vi "rsidr_core_global.vi"() -> ()   [LabVIEW 2020, in "Rohde&Schwarz CMWXP NR FR1 Measurement.lvlib"] (continued)
{"Level"=4, "Class Only"=FALSE, "Identifier"="RSCMWXPNRFR1M_ATTR_FETCH_MULTI_EVAL_MEAS_ACLR_CURRENT_RESULTS", "Descriptive Name"="Fetch Multi Eval Meas ACLR Current Results", "Data Type"=enum."RawString", "Command"="FETC:NRS:MEAS{instance}:MEV:ACLR:CURR?", "Access"=enum."Read Only", "Range Table"="", "Read Callback"="", "Write Callback"="", "Range Callback"="", "Check Callback"="", "Rngtable Callback"="", "Coerce Callback"="", "Supported Models"="", "Instrument Options"="", "Check Status Callback"="", "Flags"=0, "Help"="Returns the relative ACLR values for NR standalone, as displayed in the table below the ACLR diagram. The current values are retrieved.\n\nReturn values:  \n<Reliability>\n decimal\n\n<UTRA2neg>\n float\nACLR for the second UTRA channel with lower frequency\nDefault unit:  dB \n\n<UTRA1neg>\n float\nACLR for the first UTRA channel with lower frequency\nDefault unit:  dB \n\n<NRneg>\n float\nACLR for the first NR channel with lower frequency\nDefault unit:  dB \n\n<Carrier>\n float\nPower in the allocated NR channel\nDefault unit:  dBm \n\n<NRpos>\n float\nACLR for the first NR channel with higher frequency\nDefault unit:  dB \n\n<UTRA1pos>\n float\nACLR for the first UTRA channel with higher frequency\nDefault unit:  dB \n\n<UTRA2pos>\n float\nACLR for the second UTRA channel with higher frequency\nDefault unit:  dB\n\nAvailable Repeated Capabilities:\ninstance: i0, i1, i2, i3, i4, i5, i6, i7, i8, i9, i10, i11, i12, i13, i14, i15, i16, i17, i18, i19, i20, i21, i22, i23, i24, i25, i26, i27, i28, i29, i30, i31, i32\r\n\nRemote-control command(s):\nFETCh:NRSub:MEAS<i>:MEValuation:ACLR:CURRent?"}, {"Level"=4, "Class Only"=FALSE, "Identifier"="RSCMWXPNRFR1M_ATTR_FETCH_MULTI_EVAL_MEAS_ACLR_AVERAGE_RESULTS", "Descriptive Name"="Fetch Multi Eval Meas ACLR Average Results", "Data Type"=enum."RawString", "Command"="FETC:NRS:MEAS{instance}:MEV:ACLR:AVER?", "Access"=enum."Read Only", "Range Table"="", "Read Callback"="", "Write Callback"="", "Range Callback"="", "Check Callback"="", "Rngtable Callback"="", "Coerce Callback"="", "Supported Models"="", "Instrument Options"="", "Check Status Callback"="", "Flags"=0, "Help"="Returns the relative ACLR values for NR standalone, as displayed in the table below the ACLR diagram. The average values are retrieved.\n\nReturn values:  \n<Reliability>\n decimal\n\n<UTRA2neg>\n float\nACLR for the second UTRA channel with lower frequency\nDefault unit:  dB \n\n<UTRA1neg>\n float\nACLR for the first UTRA channel with lower frequency\nDefault unit:  dB \n\n<NRneg>\n float\nACLR for the first NR channel with lower frequency\nDefault unit:  dB \n\n<Carrier>\n float\nPower in the allocated NR channel\nDefault unit:  dBm \n\n<NRpos>\n float\nACLR for the first NR channel with higher frequency\nDefault unit:  dB \n\n<UTRA1pos>\n float\nACLR for the first UTRA channel with higher frequency\nDefault unit:  dB \n\n<UTRA2pos>\n float\nACLR for the second UTRA channel with higher frequency\nDefault unit:  dB\n\nAvailable Repeated Capabilities:\ninstance: i0, i1, i2, i3, i4, i5, i6, i7, i8, i9, i10, i11, i12, i13, i14, i15, i16, i17, i18, i19, i20, i21, i22, i23, i24, i25, i26, i27, i28, i29, i30, i31, i32\r\n\nRemote-control command(s):\nFETCh:NRSub:MEAS<i>:MEValuation:ACLR:AVERage?"}, {"Level"=4, "Class Only"=FALSE, "Identifier"="RSCMWXPNRFR1M_ATTR_QUERY_MULTI_EVAL_MEAS_ACLR_CURRENT_LIMIT_CHECK_RESULTS", "Descriptive Name"="Query Multi Eval Meas ACLR Current Limit Check Results", "Data Type"=enum."RawString", "Command"="CALC:NRS:MEAS{instance}:MEV:ACLR:CURR?", "Access"=enum."Read Only", "Range Table"="", "Read Callback"="", "Write Callback"="", "Range Callback"="", "Check Callback"="", "Rngtable Callback"="", "Coerce Callback"="", "Supported Models"="", "Instrument Options"="", "Check Status Callback"="", "Flags"=0, "Help"="Returns the limit check ACLR values for NR standalone, as displayed in the table below the ACLR diagram. The current values are used.\n\nReturn values:  \n<Reliability>\n decimal\n\n<UTRA2negLimCheck>\n limit check result\nLimit check result for the second UTRA channel with lower frequency\n\n<UTRA1negLimCheck>\n limit check result\nLimit check result for the first UTRA channel with lower frequency\n\n<NRnegLimCheck>\n limit check result\nLimit check result for the first NR channel with lower frequency\n\n<CarrierLimCheck>\n limit check result\nLimit check result for power in the allocated NR channel\n\n<NRposLimCheck>\n limit check result\nLimit check result for the first NR channel with higher frequency\n\n<UTRA1posLimCheck>\n limit check result\nLimit check result for the first UTRA channel with higher frequency\n\n<UTRA2posLimCheck>\n limit check result\nLimit check result for the second UTRA channel with higher frequency\n\nAvailable Repeated Capabilities:\ninstance: i0, i1, i2, i3, i4, i5, i6, i7, i8, i9, i10, i11, i12, i13, i14, i15, i16, i17, i18, i19, i20, i21, i22, i23, i24, i25, i26, i27, i28, i29, i30, i31, i32\r\n\nRemote-control command(s):\nCALCulate:NRSub:MEAS<i>:MEValuation:ACLR:CURRent?"}, {"Level"=4, "Class Only"=FALSE, "Identifier"="RSCMWXPNRFR1M_ATTR_QUERY_MULTI_EVAL_MEAS_ACLR_AVERAGE_LIMIT_CHECK_RESULTS", "Descriptive Name"="Query Multi Eval Meas ACLR Average Limit Check Results", "Data Type"=enum."RawString", "Command"="CALC:NRS:MEAS{instance}:MEV:ACLR:AVER?", "Access"=enum."Read Only", "Range Table"="", "Read Callback"="", "Write Callback"="", "Range Callback"="", "Check Callback"="", "Rngtable Callback"="", "Coerce Callback"="", "Supported Models"="", "Instrument Options"="", "Check Status Callback"="", "Flags"=0, "Help"="Returns the limit check ACLR values for NR standalone, as displayed in the table below the ACLR diagram. The average values are used.\n\nReturn values:  \n<Reliability>\n decimal\n\n<UTRA2negLimCheck>\n limit check result\nLimit check result for the second UTRA channel with lower frequency\n\n<UTRA1negLimCheck>\n limit check result\nLimit check result for the first UTRA channel with lower frequency\n\n<NRnegLimCheck>\n limit check result\nLimit check result for the first NR channel with lower frequency\n\n<CarrierLimCheck>\n limit check result\nLimit check result for power in the allocated NR channel\n\n<NRposLimCheck>\n limit check result\nLimit check result for the first NR channel with higher frequency\n\n<UTRA1posLimCheck>\n limit check result\nLimit check result for the first UTRA channel with higher frequency\n\n<UTRA2posLimCheck>\n limit check result\nLimit check result for the second UTRA channel with higher frequency\n\nAvailable Repeated Capabilities:\ninstance: i0, i1, i2, i3, i4, i5, i6, i7, i8, i9, i10, i11, i12, i13, i14, i15, i16, i17, i18, i19, i20, i21, i22, i23, i24, i25, i26, i27, i28, i29, i30, i31, i32\r\n\nRemote-control command(s):\nCALCulate:NRSub:MEAS<i>:MEValuation:ACLR:AVERage?"}, {"Level"=4, "Class Only"=FALSE, "Identifier"="RSCMWXPNRFR1M_ATTR_READ_MULTI_EVAL_MEAS_ACLR_ENDC_CURRENT_RESULTS", "Descriptive Name"="Read Multi Eval Meas ACLR EN-DC Current Results", "Data Type"=enum."RawString", "Command"="READ:NRS:MEAS{instance}:MEV:ACLR:ENDC:CURR?", "Access"=enum."Read Only", "Range Table"="", "Read Callback"="", "Write Callback"="", "Range Callback"="", "Check Callback"="", "Rngtable Callback"="", "Coerce Callback"="", "Supported Models"="", "Instrument Options"="", "Check Status Callback"="", "Flags"=0, "Help"="Returns the relative ACLR values for EN-DC, as displayed in the table below the ACLR diagram. The current values are retrieved.\n\nReturn values:  \n<Reliability>\n decimal\n\n<ENDCneg>\n float\nACLR for the adjacent channel with lower frequency\nDefault unit:  dB \n\n<Carrier>\n float\nPower in the allocated channel (aggregated BW)\nDefault unit:  dBm \n\n<ENDCpos>\n float\nACLR for the adjacent channel with higher frequency\nDefault unit:  dB\n\nAvailable Repeated Capabilities:\ninstance: i0, i1, i2, i3, i4, i5, i6, i7, i8, i9, i10, i11, i12, i13, i14, i15, i16, i17, i18, i19, i20, i21, i22, i23, i24, i25, i26, i27, i28, i29, i30, i31, i32\r\n\nRemote-control command(s):\nREAD:NRSub:MEAS<i>:MEValuation:ACLR:ENDC:CURRent?"}, {"Level"=4, "Class Only"=FALSE, "Identifier"="RSCMWXPNRFR1M_ATTR_READ_MULTI_EVAL_MEAS_ACLR_ENDC_AVERAGE_RESULTS", "Descriptive Name"="Read Multi Eval Meas ACLR EN-DC Average Results", "Data Type"=enum."RawString", "Command"="READ:NRS:MEAS{instance}:MEV:ACLR:ENDC:AVER?", "Access"=enum."Read Only", "Range Table"="", "Read Callback"="", "Write Callback"="", "Range Callback"="", "Check Callback"="", "Rngtable Callback"="", "Coerce Callback"="", "Supported Models"="", "Instrument Options"="", "Check Status Callback"="", "Flags"=0, "Help"="Returns the relative ACLR values for EN-DC, as displayed in the table below the ACLR diagram. The average values are retrieved.\n\nReturn values:  \n<Reliability>\n decimal\n\n<ENDCneg>\n float\nACLR for the adjacent channel with lower frequency\nDefault unit:  dB \n\n<Carrier>\n float\nPower in the allocated channel (aggregated BW)\nDefault unit:  dBm \n\n<ENDCpos>\n float\nACLR for the adjacent channel with higher frequency\nDefault unit:  dB\n\nAvailable Repeated Capabilities:\ninstance: i0, i1, i2, i3, i4, i5, i6, i7, i8, i9, i10, i11, i12, i13, i14, i15, i16, i17, i18, i19, i20, i21, i22, i23, i24, i25, i26, i27, i28, i29, i30, i31, i32\r\n\nRemote-control command(s):\nREAD:NRSub:MEAS<i>:MEValuation:ACLR:ENDC:AVERage?"}, {"Level"=4, "Class Only"=FALSE, "Identifier"="RSCMWXPNRFR1M_ATTR_FETCH_MULTI_EVAL_MEAS_ACLR_ENDC_CURRENT_RESULTS", "Descriptive Name"="Fetch Multi Eval Meas ACLR EN-DC Current Results", "Data Type"=enum."RawString", "Command"="FETC:NRS:MEAS{instance}:MEV:ACLR:ENDC:CURR?", "Access"=enum."Read Only", "Range Table"="", "Read Callback"="", "Write Callback"="", "Range Callback"="", "Check Callback"="", "Rngtable Callback"="", "Coerce Callback"="", "Supported Models"="", "Instrument Options"="", "Check Status Callback"="", "Flags"=0, "Help"="Returns the relative ACLR values for EN-DC, as displayed in the table below the ACLR diagram. The current values are retrieved.\n\nReturn values:  \n<Reliability>\n decimal\n\n<ENDCneg>\n float\nACLR for the adjacent channel with lower frequency\nDefault unit:  dB \n\n<Carrier>\n float\nPower in the allocated channel (aggregated BW)\nDefault unit:  dBm \n\n<ENDCpos>\n float\nACLR for the adjacent channel with higher frequency\nDefault unit:  dB\n\nAvailable Repeated Capabilities:\ninstance: i0, i1, i2, i3, i4, i5, i6, i7, i8, i9, i10, i11, i12, i13, i14, i15, i16, i17, i18, i19, i20, i21, i22, i23, i24, i25, i26, i27, i28, i29, i30, i31, i32\r\n\nRemote-control command(s):\nFETCh:NRSub:MEAS<i>:MEValuation:ACLR:ENDC:CURRent?"}, {"Level"=4, "Class Only"=FALSE, "Identifier"="RSCMWXPNRFR1M_ATTR_FETCH_MULTI_EVAL_MEAS_ACLR_ENDC_AVERAGE_RESULTS", "Descriptive Name"="Fetch Multi Eval Meas ACLR EN-DC Average Results", "Data Type"=enum."RawString", "Command"="FETC:NRS:MEAS{instance}:MEV:ACLR:ENDC:AVER?", "Access"=enum."Read Only", "Range Table"="", "Read Callback"="", "Write Callback"="", "Range Callback"="", "Check Callback"="", "Rngtable Callback"="", "Coerce Callback"="", "Supported Models"="", "Instrument Options"="", "Check Status Callback"="", "Flags"=0, "Help"="Returns the relative ACLR values for EN-DC, as displayed in the table below the ACLR diagram. The average values are retrieved.\n\nReturn values:  \n<Reliability>\n decimal\n\n<ENDCneg>\n float\nACLR for the adjacent channel with lower frequency\nDefault unit:  dB \n\n<Carrier>\n float\nPower in the allocated channel (aggregated BW)\nDefault unit:  dBm \n\n<ENDCpos>\n float\nACLR for the adjacent channel with higher frequency\nDefault unit:  dB\n\nAvailable Repeated Capabilities:\ninstance: i0, i1, i2, i3, i4, i5, i6, i7, i8, i9, i10, i11, i12, i13, i14, i15, i16, i17, i18, i19, i20, i21, i22, i23, i24, i25, i26, i27, i28, i29, i30, i31, i32\r\n\nRemote-control command(s):\nFETCh:NRSub:MEAS<i>:MEValuation:ACLR:ENDC:AVERage?"}, {"Level"=4, "Class Only"=FALSE, "Identifier"="RSCMWXPNRFR1M_ATTR_QUERY_MULTI_EVAL_MEAS_ACLR_ENDC_CURRENT_LIMIT_CHECK_RESULTS", "Descriptive Name"="Query Multi Eval Meas ACLR EN-DC Current Limit Check Results", "Data Type"=enum."RawString", "Command"="CALC:NRS:MEAS{instance}:MEV:ACLR:ENDC:CURR?", "Access"=enum."Read Only", "Range Table"="", "Read Callback"="", "Write Callback"="", "Range Callback"="", "Check Callback"="", "Rngtable Callback"="", "Coerce Callback"="", "Supported Models"="", "Instrument Options"="", "Check Status Callback"="", "Flags"=0, "Help"="Returns the ACLR limit check values for EN-DC, as displayed in the table below the ACLR diagram. The current values are used.\n\nReturn values:  \n<Reliability>\n decimal\n\n<ENDCnegLimCheck>\n limit check result\nLimit check result for the adjacent channel with lower frequency\n\n<CarrierLimCheck>\n limit check result\nLimit check result for power in the allocated channel (aggregated BW)\n\n<ENDCposLimCheck>\n limit check result\nLimit check result for the adjacent channel with higher frequency\n\nAvailable Repeated Capabilities:\ninstance: i0, i1, i2, i3, i4, i5, i6, i7, i8, i9, i10, i11, i12, i13, i14, i15, i16, i17, i18, i19, i20, i21, i22, i23, i24, i25, i26, i27, i28, i29, i30, i31, i32\r\n\nRemote-control command(s):\nCALCulate:NRSub:MEAS<i>:MEValuation:ACLR:ENDC:CURRent?"}, {"Level"=4, "Class Only"=FALSE, "Identifier"="RSCMWXPNRFR1M_ATTR_QUERY_MULTI_EVAL_MEAS_ACLR_ENDC_AVERAGE_LIMIT_CHECK_RESULTS", "Descriptive Name"="Query Multi Eval Meas ACLR EN-DC Average Limit Check Results", "Data Type"=enum."RawString", "Command"="CALC:NRS:MEAS{instance}:MEV:ACLR:ENDC:AVER?", "Access"=enum."Read Only", "Range Table"="", "Read Callback"="", "Write Callback"="", "Range Callback"="", "Check Callback"="", "Rngtable Callback"="", "Coerce Callback"="", "Supported Models"="", "Instrument Options"="", "Check Status Callback"="", "Flags"=0, "Help"="Returns the ACLR limit check values for EN-DC, as displayed in the table below the ACLR diagram. The current values are used.\n\nReturn values:  \n<Reliability>\n decimal\n\n<ENDCnegLimCheck>\n limit check result\nLimit check result for the adjacent channel with lower frequency\n\n<CarrierLimCheck>\n limit check result\nLimit check result for power in the allocated channel (aggregated BW)\n\n<ENDCposLimCheck>\n limit check result\nLimit check result for the adjacent channel with higher frequency\n\nAvailable Repeated Capabilities:\ninstance: i0, i1, i2, i3, i4, i5, i6, i7, i8, i9, i10, i11, i12, i13, i14, i15, i16, i17, i18, i19, i20, i21, i22, i23, i24, i25, i26, i27, i28, i29, i30, i31, i32\r\n\nRemote-control command(s):\nCALCulate:NRSub:MEAS<i>:MEValuation:ACLR:ENDC:AVERage?"}, {"Level"=3, "Class Only"=TRUE, "Identifier"="", "Descriptive Name"="IQ Constellation", "Data Type"=enum."ViInt32", "Command"="", "Access"=enum."Read Only", "Range Table"="", "Read Callback"="", "Write Callback"="", "Range Callback"="", "Check Callback"="", "Rngtable Callback"="", "Coerce Callback"="", "Supported Models"="", "Instrument Options"="", "Check Status Callback"="", "Flags"=0, "Help"="This class contains commands that return the contents of the I/Q constellation diagram."}, {"Level"=4, "Class Only"=FALSE, "Identifier"="RSCMWXPNRFR1M_ATTR_FETCH_MULTI_EVAL_MEAS_TRACE_IQ_CONSTELLATION_LOW_RESULTS", "Descriptive Name"="Fetch Multi Eval Meas Trace IQ Constellation Low Results", "Data Type"=enum."RawString", "Command"="FETC:NRS:MEAS{instance}:MEV:TRAC:IQ:LOW?", "Access"=enum."Read Only", "Range Table"="", "Read Callback"="", "Write Callback"="", "Range Callback"="", "Check Callback"="", "Rngtable Callback"="", "Coerce Callback"="", "Supported Models"="", "Instrument Options"="", "Check Status Callback"="", "Flags"=0, "Help"="Returns the results in the I/Q constellation diagram for low EVM window position.\n\nThere is one pair of values per modulation symbol. The results are returned in the following order:\n<Reliability>, {<IPhase>, <QPhase>}symbol 1, ..., {<IPhase>, <QPhase>}symbol n\n\nReturn values:  \n<Reliability>\n decimal\n\n<IPhase>\n float\nNormalized I amplitude\n\n<QPhase>\n float\nNormalized Q amplitude\n\nAvailable Repeated Capabilities:\ninstance: i0, i1, i2, i3, i4, i5, i6, i7, i8, i9, i10, i11, i12, i13, i14, i15, i16, i17, i18, i19, i20, i21, i22, i23, i24, i25, i26, i27, i28, i29, i30, i31, i32\r\n\nRemote-control command(s):\nFETCh:NRSub:MEAS<i>:MEValuation:TRACe:IQ:LOW?"}, {"Level"=4, "Class Only"=FALSE, "Identifier"="RSCMWXPNRFR1M_ATTR_FETCH_MULTI_EVAL_MEAS_TRACE_IQ_CONSTELLATION_HIGH_RESULTS", "Descriptive Name"="Fetch Multi Eval Meas Trace IQ Constellation High Results", "Data Type"=enum."RawString", "Command"="FETC:NRS:MEAS{instance}:MEV:TRAC:IQ:HIGH?", "Access"=enum."Read Only", "Range Table"="", "Read Callback"="", "Write Callback"="", "Range Callback"="", "Check Callback"="", "Rngtable Callback"="", "Coerce Callback"="", "Supported Models"="", "Instrument Options"="", "Check Status Callback"="", "Flags"=0, "Help"="Returns the results in the I/Q constellation diagram for high EVM window position.\n\nThere is one pair of values per modulation symbol. The results are returned in the following order:\n<Reliability>, {<IPhase>, <QPhase>}symbol 1, ..., {<IPhase>, <QPhase>}symbol n\n\nReturn values:  \n<Reliability>\n decimal\n\n<IPhase>\n float\nNormalized I amplitude\n\n<QPhase>\n float\nNormalized Q amplitude\n\nAvailable Repeated Capabilities:\ninstance: i0, i1, i2, i3, i4, i5, i6, i7, i8, i9, i10, i11, i12, i13, i14, i15, i16, i17, i18, i19, i20, i21, i22, i23, i24, i25, i26, i27, i28, i29, i30, i31, i32\r\n\nRemote-control command(s):\nFETCh:NRSub:MEAS<i>:MEValuation:TRACe:IQ:HIGH?"}, {"Level"=3, "Class Only"=TRUE, "Identifier"="", "Descriptive Name"="Modulation", "Data Type"=enum."ViInt32", "Command"="", "Access"=enum."Read Only", "Range Table"="", "Read Callback"="", "Write Callback"="", "Range Callback"="", "Check Callback"="", "Rngtable Callback"="", "Coerce Callback"="", "Supported Models"="", "Instrument Options"="", "Check Status Callback"="", "Flags"=0, "Help"="The commands in this class return the statistical modulation results."}, {"Level"=4, "Class Only"=FALSE, "Identifier"="RSCMWXPNRFR1M_ATTR_READ_MULTI_EVAL_MEAS_MODULATION_CURRENT_RESULTS", "Descriptive Name"="Read Multi Eval Meas Modulation Current Results", "Data Type"=enum."RawString", "Command"="READ:NRS:MEAS{instance}:MEV:MOD:CURR?", "Access"=enum."Read Only", "Range Table"="", "Read Callback"="", "Write Callback"="", "Range Callback"="", "Check Callback"="", "Rngtable Callback"="", "Coerce Callback"="", "Supported Models"="", "Instrument Options"="", "Check Status Callback"="", "Flags"=0, "Help"="Return the current single value results.\n\nReturn values:  \n<1_Reliability>\n decimal\n\n<2_OutOfTol>\n decimal\nOut of tolerance result, i.e. percentage of measurement intervals of the statistic count for modulation measurements exceeding the specified modulation limits.\nDefault unit:  % \n\n<3_EVM_RMSlow>\n float\nEVM RMS value, low EVM window position\nDefault unit:  % \n\n<4_EVM_RMShigh>\n float\nEVM RMS value, high EVM window position\nDefault unit:  % \n\n<5_EVMpeakLow>\n float\nEVM peak value, low EVM window position\nDefault unit:  % \n\n<6_EVMpeakHigh>\n float\nEVM peak value, high EVM window position\nDefault unit:  % \n\n<7_MErr_RMSlow>\n float\nMagnitude error RMS value, low EVM window position\nDefault unit:  % \n\n<8_MErr_RMShigh>\n float\nMagnitude error RMS value, high EVM window position\nDefault unit:  % \n\n<9_MErrPeakLow>\n float\nMagnitude error peak value, low EVM window position\nDefault unit:  % \n\n<10_MErrPeakHigh>\n float\nMagnitude error peak value, high EVM window position\nDefault unit:  % \n\n<11_PErr_RMSlow>\n float\nPhase error RMS value, low EVM window position\nDefault unit:  deg \n\n<12_PErr_RMSh>\n float\nPhase error RMS value, high EVM window position\nDefault unit:  deg \n\n<13_PErrPeakLow>\n float\nPhase error peak value, low EVM window position\nDefault unit:  deg \n\n<14_PErrPeakHigh>\n float\nPhase error peak value, high EVM window position\nDefault unit:  deg \n\n<15_IQoffset>\n float\nI/Q origin offset\nDefault unit:  dBc \n\n<16_FreqError>\n float\nCarrier frequency error\nDefault unit:  Hz \n\n<17_TimingError>\n float\nTransmit time error\nDefault unit:  Ts (basic time unit) \n\n<18_TXpower>\n float\nUser equipment power\nDefault unit:  dBm \n\n<19_PeakPower>\n float\nUser equipment peak power\nDefault unit:  dBm \n\n<20_RBpower>\n float\nRB power\nDefault unit:  dBm \n\n<21_EVM_DMRSl>\n float\nEVM DMRS value, low EVM window position\nDefault unit:  % \n\n<22_EVM_DMRSh>\n float\nEVM DMRS value, high EVM window position\nDefault unit:  % \n\n<23_MErr_DMRSl>\n float\nMagnitude error DMRS value, low EVM window position\nDefault unit:  % \n\n<24_MErr_DMRSh>\n float\nMagnitude error DMRS value, high EVM window position\nDefault unit:  % \n\n<25_PErr_DMRS>\n float\nPhase error DMRS value, low EVM window position\nDefault unit:  deg \n\n<26_PErr_DMRSh>\n float\nPhase error DMRS value, high EVM window position\nDefault unit:  deg \n\n<27_FreqErrorPpm>\n float\nCarrier frequency error in ppm\nDefault unit:  ppm \n\n<28_SampleClockE>\n float\nSample clock error\nDefault unit:  ppm\n\nAvailable Repeated Capabilities:\ninstance: i0, i1, i2, i3, i4, i5, i6, i7, i8, i9, i10, i11, i12, i13, i14, i15, i16, i17, i18, i19, i20, i21, i22, i23, i24, i25, i26, i27, i28, i29, i30, i31, i32\r\n\nRemote-control command(s):\nREAD:NRSub:MEAS<i>:MEValuation:MODulation:CURRent?"}, {"Level"=4, "Class Only"=FALSE, "Identifier"="RSCMWXPNRFR1M_ATTR_READ_MULTI_EVAL_MEAS_MODULATION_AVERAGE_RESULTS", "Descriptive Name"="Read Multi Eval Meas Modulation Average Results", "Data Type"=enum."RawString", "Command"="READ:NRS:MEAS{instance}:MEV:MOD:AVER?", "Access"=enum."Read Only", "Range Table"="", "Read Callback"="", "Write Callback"="", "Range Callback"="", "Check Callback"="", "Rngtable Callback"="", "Coerce Callback"="", "Supported Models"="", "Instrument Options"="", "Check Status Callback"="", "Flags"=0, "Help"="Return the average single value results.\n\nReturn values:  \n<1_Reliability>\n decimal\n\n<2_OutOfTol>\n decimal\nOut of tolerance result, i.e. percentage of measurement intervals of the statistic count for modulation measurements exceeding the specified modulation limits.\nDefault unit:  % \n\n<3_EVM_RMSlow>\n float\nEVM RMS value, low EVM window position\nDefault unit:  % \n\n<4_EVM_RMShigh>\n float\nEVM RMS value, high EVM window position\nDefault unit:  % \n\n<5_EVMpeakLow>\n float\nEVM peak value, low EVM window position\nDefault unit:  % \n\n<6_EVMpeakHigh>\n float\nEVM peak value, high EVM window position\nDefault unit:  % \n\n<7_MErr_RMSlow>\n float\nMagnitude error RMS value, low EVM window position\nDefault unit:  % \n\n<8_MErr_RMShigh>\n float\nMagnitude error RMS value, high EVM window position\nDefault unit:  % \n\n<9_MErrPeakLow>\n float\nMagnitude error peak value, low EVM window position\nDefault unit:  % \n\n<10_MErrPeakHigh>\n float\nMagnitude error peak value, high EVM window position\nDefault unit:  % \n\n<11_PErr_RMSlow>\n float\nPhase error RMS value, low EVM window position\nDefault unit:  deg \n\n<12_PErr_RMSh>\n float\nPhase error RMS value, high EVM window position\nDefault unit:  deg \n\n<13_PErrPeakLow>\n float\nPhase error peak value, low EVM window position\nDefault unit:  deg \n\n<14_PErrPeakHigh>\n float\nPhase error peak value, high EVM window position\nDefault unit:  deg \n\n<15_IQoffset>\n float\nI/Q origin offset\nDefault unit:  dBc \n\n<16_FreqError>\n float\nCarrier frequency error\nDefault unit:  Hz \n\n<17_TimingError>\n float\nTransmit time error\nDefault unit:  Ts (basic time unit) \n\n<18_TXpower>\n float\nUser equipment power\nDefault unit:  dBm \n\n<19_PeakPower>\n float\nUser equipment peak power\nDefault unit:  dBm \n\n<20_RBpower>\n float\nRB power\nDefault unit:  dBm \n\n<21_EVM_DMRSl>\n float\nEVM DMRS value, low EVM window position\nDefault unit:  % \n\n<22_EVM_DMRSh>\n float\nEVM DMRS value, high EVM window position\nDefault unit:  % \n\n<23_MErr_DMRSl>\n float\nMagnitude error DMRS value, low EVM window position\nDefault unit:  % \n\n<24_MErr_DMRSh>\n float\nMagnitude error DMRS value, high EVM window position\nDefault unit:  % \n\n<25_PErr_DMRS>\n float\nPhase error DMRS value, low EVM window position\nDefault unit:  deg \n\n<26_PErr_DMRSh>\n float\nPhase error DMRS value, high EVM window position\nDefault unit:  deg \n\n<27_FreqErrorPpm>\n float\nCarrier frequency error in ppm\nDefault unit:  ppm \n\n<28_SampleClockE>\n float\nSample clock error\nDefault unit:  ppm\n\nAvailable Repeated Capabilities:\ninstance: i0, i1, i2, i3, i4, i5, i6, i7, i8, i9, i10, i11, i12, i13, i14, i15, i16, i17, i18, i19, i20, i21, i22, i23, i24, i25, i26, i27, i28, i29, i30, i31, i32\r\n\nRemote-control command(s):\nREAD:NRSub:MEAS<i>:MEValuation:MODulation:AVERage?"}, {"Level"=4, "Class Only"=FALSE, "Identifier"="RSCMWXPNRFR1M_ATTR_READ_MULTI_EVAL_MEAS_MODULATION_STANDARD_DEVIATION_RESULTS", "Descriptive Name"="Read Multi Eval Meas Modulation Standard Deviation Results", "Data Type"=enum."RawString", "Command"="READ:NRS:MEAS{instance}:MEV:MOD:SDEV?", "Access"=enum."Read Only", "Range Table"="", "Read Callback"="", "Write Callback"="", "Range Callback"="", "Check Callback"="", "Rngtable Callback"="", "Coerce Callback"="", "Supported Models"="", "Instrument Options"="", "Check Status Callback"="", "Flags"=0, "Help"="Return the standard deviation single value results.\n\nReturn values:  \n<1_Reliability>\n decimal\n\n<2_OutOfTol>\n decimal\nOut of tolerance result, i.e. percentage of measurement intervals of the statistic count for modulation measurements exceeding the specified modulation limits.\nDefault unit:  % \n\n<3_EVM_RMSlow>\n float\nEVM RMS value, low EVM window position\nDefault unit:  % \n\n<4_EVM_RMShigh>\n float\nEVM RMS value, high EVM window position\nDefault unit:  % \n\n<5_EVMpeakLow>\n float\nEVM peak value, low EVM window position\nDefault unit:  % \n\n<6_EVMpeakHigh>\n float\nEVM peak value, high EVM window position\nDefault unit:  % \n\n<7_MErr_RMSlow>\n float\nMagnitude error RMS value, low EVM window position\nDefault unit:  % \n\n<8_MErr_RMShigh>\n float\nMagnitude error RMS value, high EVM window position\nDefault unit:  % \n\n<9_MErrPeakLow>\n float\nMagnitude error peak value, low EVM window position\nDefault unit:  % \n\n<10_MErrPeakHigh>\n float\nMagnitude error peak value, high EVM window position\nDefault unit:  % \n\n<11_PErr_RMSlow>\n float\nPhase error RMS value, low EVM window position\nDefault unit:  deg \n\n<12_PErr_RMSh>\n float\nPhase error RMS value, high EVM window position\nDefault unit:  deg \n\n<13_PErrPeakLow>\n float\nPhase error peak value, low EVM window position\nDefault unit:  deg \n\n<14_PErrPeakHigh>\n float\nPhase error peak value, high EVM window position\nDefault unit:  deg \n\n<15_IQoffset>\n float\nI/Q origin offset\nDefault unit:  dBc \n\n<16_FreqError>\n float\nCarrier frequency error\nDefault unit:  Hz \n\n<17_TimingError>\n float\nTransmit time error\nDefault unit:  Ts (basic time unit) \n\n<18_TXpower>\n float\nUser equipment power\nDefault unit:  dBm \n\n<19_PeakPower>\n float\nUser equipment peak power\nDefault unit:  dBm \n\n<20_RBpower>\n float\nRB power\nDefault unit:  dBm \n\n<21_EVM_DMRSl>\n float\nEVM DMRS value, low EVM window position\nDefault unit:  % \n\n<22_EVM_DMRSh>\n float\nEVM DMRS value, high EVM window position\nDefault unit:  % \n\n<23_MErr_DMRSl>\n float\nMagnitude error DMRS value, low EVM window position\nDefault unit:  % \n\n<24_MErr_DMRSh>\n float\nMagnitude error DMRS value, high EVM window position\nDefault unit:  % \n\n<25_PErr_DMRS>\n float\nPhase error DMRS value, low EVM window position\nDefault unit:  deg \n\n<26_PErr_DMRSh>\n float\nPhase error DMRS value, high EVM window position\nDefault unit:  deg \n\n<27_FreqErrorPpm>\n float\nCarrier frequency error in ppm\nDefault unit:  ppm \n\n<28_SampleClockE>\n float\nSample clock error\nDefault unit:  ppm\n\nAvailable Repeated Capabilities:\ninstance: i0, i1, i2, i3, i4, i5, i6, i7, i8, i9, i10, i11, i12, i13, i14, i15, i16, i17, i18, i19, i20, i21, i22, i23, i24, i25, i26, i27, i28, i29, i30, i31, i32\r\n\nRemote-control command(s):\nREAD:NRSub:MEAS<i>:MEValuation:MODulation:SDEViation?"}, {"Level"=4, "Class Only"=FALSE, "Identifier"="RSCMWXPNRFR1M_ATTR_FETCH_MULTI_EVAL_MEAS_MODULATION_CURRENT_RESULTS", "Descriptive Name"="Fetch Multi Eval Meas Modulation Current Results", "Data Type"=enum."RawString", "Command"="FETC:NRS:MEAS{instance}:MEV:MOD:CURR?", "Access"=enum."Read Only", "Range Table"="", "Read Callback"="", "Write Callback"="", "Range Callback"="", "Check Callback"="", "Rngtable Callback"="", "Coerce Callback"="", "Supported Models"="", "Instrument Options"="", "Check Status Callback"="", "Flags"=0, "Help"="Return the current single value results.\n\nReturn values:  \n<1_Reliability>\n decimal\n\n<2_OutOfTol>\n decimal\nOut of tolerance result, i.e. percentage of measurement intervals of the statistic count for modulation measurements exceeding the specified modulation limits.\nDefault unit:  % \n\n<3_EVM_RMSlow>\n float\nEVM RMS value, low EVM window position\nDefault unit:  % \n\n<4_EVM_RMShigh>\n float\nEVM RMS value, high EVM window position\nDefault unit:  % \n\n<5_EVMpeakLow>\n float\nEVM peak value, low EVM window position\nDefault unit:  % \n\n<6_EVMpeakHigh>\n float\nEVM peak value, high EVM window position\nDefault unit:  % \n\n<7_MErr_RMSlow>\n float\nMagnitude error RMS value, low EVM window position\nDefault unit:  % \n\n<8_MErr_RMShigh>\n float\nMagnitude error RMS value, high EVM window position\nDefault unit:  % \n\n<9_MErrPeakLow>\n float\nMagnitude error peak value, low EVM window position\nDefault unit:  % \n\n<10_MErrPeakHigh>\n float\nMagnitude error peak value, high EVM window position\nDefault unit:  % \n\n<11_PErr_RMSlow>\n float\nPhase error RMS value, low EVM window position\nDefault unit:  deg \n\n<12_PErr_RMSh>\n float\nPhase error RMS value, high EVM window position\nDefault unit:  deg \n\n<13_PErrPeakLow>\n float\nPhase error peak value, low EVM window position\nDefault unit:  deg \n\n<14_PErrPeakHigh>\n float\nPhase error peak value, high EVM window position\nDefault unit:  deg \n\n<15_IQoffset>\n float\nI/Q origin offset\nDefault unit:  dBc \n\n<16_FreqError>\n float\nCarrier frequency error\nDefault unit:  Hz \n\n<17_TimingError>\n float\nTransmit time error\nDefault unit:  Ts (basic time unit) \n\n<18_TXpower>\n float\nUser equipment power\nDefault unit:  dBm \n\n<19_PeakPower>\n float\nUser equipment peak power\nDefault unit:  dBm \n\n<20_RBpower>\n float\nRB power\nDefault unit:  dBm \n\n<21_EVM_DMRSl>\n float\nEVM DMRS value, low EVM window position\nDefault unit:  % \n\n<22_EVM_DMRSh>\n float\nEVM DMRS value, high EVM window position\nDefault unit:  % \n\n<23_MErr_DMRSl>\n float\nMagnitude error DMRS value, low EVM window position\nDefault unit:  % \n\n<24_MErr_DMRSh>\n float\nMagnitude error DMRS value, high EVM window position\nDefault unit:  % \n\n<25_PErr_DMRS>\n float\nPhase error DMRS value, low EVM window position\nDefault unit:  deg \n\n<26_PErr_DMRSh>\n float\nPhase error DMRS value, high EVM window position\nDefault unit:  deg \n\n<27_FreqErrorPpm>\n float\nCarrier frequency error in ppm\nDefault unit:  ppm \n\n<28_SampleClockE>\n float\nSample clock error\nDefault unit:  ppm\n\nAvailable Repeated Capabilities:\ninstance: i0, i1, i2, i3, i4, i5, i6, i7, i8, i9, i10, i11, i12, i13, i14, i15, i16, i17, i18, i19, i20, i21, i22, i23, i24, i25, i26, i27, i28, i29, i30, i31, i32\r\n\nRemote-control command(s):\nFETCh:NRSub:MEAS<i>:MEValuation:MODulation:CURRent?"}, {"Level"=4, "Class Only"=FALSE, "Identifier"="RSCMWXPNRFR1M_ATTR_FETCH_MULTI_EVAL_MEAS_MODULATION_AVERAGE_RESULTS", "Descriptive Name"="Fetch Multi Eval Meas Modulation Average Results", "Data Type"=enum."RawString", "Command"="FETC:NRS:MEAS{instance}:MEV:MOD:AVER?", "Access"=enum."Read Only", "Range Table"="", "Read Callback"="", "Write Callback"="", "Range Callback"="", "Check Callback"="", "Rngtable Callback"="", "Coerce Callback"="", "Supported Models"="", "Instrument Options"="", "Check Status Callback"="", "Flags"=0, "Help"="Return the average single value results.\n\nReturn values:  \n<1_Reliability>\n decimal\n\n<2_OutOfTol>\n decimal\nOut of tolerance result, i.e. percentage of measurement intervals of the statistic count for modulation measurements exceeding the specified modulation limits.\nDefault unit:  % \n\n<3_EVM_RMSlow>\n float\nEVM RMS value, low EVM window position\nDefault unit:  % \n\n<4_EVM_RMShigh>\n float\nEVM RMS value, high EVM window position\nDefault unit:  % \n\n<5_EVMpeakLow>\n float\nEVM peak value, low EVM window position\nDefault unit:  % \n\n<6_EVMpeakHigh>\n float\nEVM peak value, high EVM window position\nDefault unit:  % \n\n<7_MErr_RMSlow>\n float\nMagnitude error RMS value, low EVM window position\nDefault unit:  % \n\n<8_MErr_RMShigh>\n float\nMagnitude error RMS value, high EVM window position\nDefault unit:  % \n\n<9_MErrPeakLow>\n float\nMagnitude error peak value, low EVM window position\nDefault unit:  % \n\n<10_MErrPeakHigh>\n float\nMagnitude error peak value, high EVM window position\nDefault unit:  % \n\n<11_PErr_RMSlow>\n float\nPhase error RMS value, low EVM window position\nDefault unit:  deg \n\n<12_PErr_RMSh>\n float\nPhase error RMS value, high EVM window position\nDefault unit:  deg \n\n<13_PErrPeakLow>\n float\nPhase error peak value, low EVM window position\nDefault unit:  deg \n\n<14_PErrPeakHigh>\n float\nPhase error peak value, high EVM window position\nDefault unit:  deg \n\n<15_IQoffset>\n float\nI/Q origin offset\nDefault unit:  dBc \n\n<16_FreqError>\n float\nCarrier frequency error\nDefault unit:  Hz \n\n<17_TimingError>\n float\nTransmit time error\nDefault unit:  Ts (basic time unit) \n\n<18_TXpower>\n float\nUser equipment power\nDefault unit:  dBm \n\n<19_PeakPower>\n float\nUser equipment peak power\nDefault unit:  dBm \n\n<20_RBpower>\n float\nRB power\nDefault unit:  dBm \n\n<21_EVM_DMRSl>\n float\nEVM DMRS value, low EVM window position\nDefault unit:  % \n\n<22_EVM_DMRSh>\n float\nEVM DMRS value, high EVM window position\nDefault unit:  % \n\n<23_MErr_DMRSl>\n float\nMagnitude error DMRS value, low EVM window position\nDefault unit:  % \n\n<24_MErr_DMRSh>\n float\nMagnitude error DMRS value, high EVM window position\nDefault unit:  % \n\n<25_PErr_DMRS>\n float\nPhase error DMRS value, low EVM window position\nDefault unit:  deg \n\n<26_PErr_DMRSh>\n float\nPhase error DMRS value, high EVM window position\nDefault unit:  deg \n\n<27_FreqErrorPpm>\n float\nCarrier frequency error in ppm\nDefault unit:  ppm \n\n<28_SampleClockE>\n float\nSample clock error\nDefault unit:  ppm\n\nAvailable Repeated Capabilities:\ninstance: i0, i1, i2, i3, i4, i5, i6, i7, i8, i9, i10, i11, i12, i13, i14, i15, i16, i17, i18, i19, i20, i21, i22, i23, i24, i25, i26, i27, i28, i29, i30, i31, i32\r\n\nRemote-control command(s):\nFETCh:NRSub:MEAS<i>:MEValuation:MODulation:AVERage?"}, {"Level"=4, "Class Only"=FALSE, "Identifier"="RSCMWXPNRFR1M_ATTR_FETCH_MULTI_EVAL_MEAS_MODULATION_STANDARD_DEVIATION_RESULTS", "Descriptive Name"="Fetch Multi Eval Meas Modulation Standard Deviation Results", "Data Type"=enum."RawString", "Command"="FETC:NRS:MEAS{instance}:MEV:MOD:SDEV?", "Access"=enum."Read Only", "Range Table"="", "Read Callback"="", "Write Callback"="", "Range Callback"="", "Check Callback"="", "Rngtable Callback"="", "Coerce Callback"="", "Supported Models"="", "Instrument Options"="", "Check Status Callback"="", "Flags"=0, "Help"="Return the standard deviation single value results.\n\nReturn values:  \n<1_Reliability>\n decimal\n\n<2_OutOfTol>\n decimal\nOut of tolerance result, i.e. percentage of measurement intervals of the statistic count for modulation measurements exceeding the specified modulation limits.\nDefault unit:  % \n\n<3_EVM_RMSlow>\n float\nEVM RMS value, low EVM window position\nDefault unit:  % \n\n<4_EVM_RMShigh>\n float\nEVM RMS value, high EVM window position\nDefault unit:  % \n\n<5_EVMpeakLow>\n float\nEVM peak value, low EVM window position\nDefault unit:  % \n\n<6_EVMpeakHigh>\n float\nEVM peak value, high EVM window position\nDefault unit:  % \n\n<7_MErr_RMSlow>\n float\nMagnitude error RMS value, low EVM window position\nDefault unit:  % \n\n<8_MErr_RMShigh>\n float\nMagnitude error RMS value, high EVM window position\nDefault unit:  % \n\n<9_MErrPeakLow>\n float\nMagnitude error peak value, low EVM window position\nDefault unit:  % \n\n<10_MErrPeakHigh>\n float\nMagnitude error peak value, high EVM window position\nDefault unit:  % \n\n<11_PErr_RMSlow>\n float\nPhase error RMS value, low EVM window position\nDefault unit:  deg \n\n<12_PErr_RMSh>\n float\nPhase error RMS value, high EVM window position\nDefault unit:  deg \n\n<13_PErrPeakLow>\n float\nPhase error peak value, low EVM window position\nDefault unit:  deg \n\n<14_PErrPeakHigh>\n float\nPhase error peak value, high EVM window position\nDefault unit:  deg \n\n<15_IQoffset>\n float\nI/Q origin offset\nDefault unit:  dBc \n\n<16_FreqError>\n float\nCarrier frequency error\nDefault unit:  Hz \n\n<17_TimingError>\n float\nTransmit time error\nDefault unit:  Ts (basic time unit) \n\n<18_TXpower>\n float\nUser equipment power\nDefault unit:  dBm \n\n<19_PeakPower>\n float\nUser equipment peak power\nDefault unit:  dBm \n\n<20_RBpower>\n float\nRB power\nDefault unit:  dBm \n\n<21_EVM_DMRSl>\n float\nEVM DMRS value, low EVM window position\nDefault unit:  % \n\n<22_EVM_DMRSh>\n float\nEVM DMRS value, high EVM window position\nDefault unit:  % \n\n<23_MErr_DMRSl>\n float\nMagnitude error DMRS value, low EVM window position\nDefault unit:  % \n\n<24_MErr_DMRSh>\n float\nMagnitude error DMRS value, high EVM window position\nDefault unit:  % \n\n<25_PErr_DMRS>\n float\nPhase error DMRS value, low EVM window position\nDefault unit:  deg \n\n<26_PErr_DMRSh>\n float\nPhase error DMRS value, high EVM window position\nDefault unit:  deg \n\n<27_FreqErrorPpm>\n float\nCarrier frequency error in ppm\nDefault unit:  ppm \n\n<28_SampleClockE>\n float\nSample clock error\nDefault unit:  ppm\n\nAvailable Repeated Capabilities:\ninstance: i0, i1, i2, i3, i4, i5, i6, i7, i8, i9, i10, i11, i12, i13, i14, i15, i16, i17, i18, i19, i20, i21, i22, i23, i24, i25, i26, i27, i28, i29, i30, i31, i32\r\n\nRemote-control command(s):\nFETCh:NRSub:MEAS<i>:MEValuation:MODulation:SDEViation?"}, {"Level"=4, "Class Only"=FALSE, "Identifier"="RSCMWXPNRFR1M_ATTR_QUERY_MULTI_EVAL_MEAS_MODULATION_CURRENT_LIMIT_CHECK_RESULTS", "Descriptive Name"="Query Multi Eval Meas Modulation Current Limit Check Results", "Data Type"=enum."RawString", "Command"="CALC:NRS:MEAS{instance}:MEV:MOD:CURR?", "Access"=enum."Read Only", "Range Table"="", "Read Callback"="", "Write Callback"="", "Range Callback"="", "Check Callback"="", "Rngtable Callback"="", "Coerce Callback"="", "Supported Models"="", "Instrument Options"="", "Check Status Callback"="", "Flags"=0, "Help"="Return the current single value limit check results.\n\nReturn values:  \n<1_Reliability>\n decimal\n\n<2_OutOfTol>\n decimal\nOut of tolerance result, i.e. percentage of measurement intervals of the statistic count for modulation measurements exceeding the specified modulation limits.\n\n<3_EVM_RMSlowLimCheck>\n limit check result\nEVM RMS value, low EVM window position\n\n<4_EVM_RMShighLimCheck>\n limit check result\nEVM RMS value, high EVM window position\n\n<5_EVMpeakLowLimCheck>\n limit check result\nEVM peak value, low EVM window position\n\n<6_EVMpeakHighLimCheck>\n limit check result\nEVM peak value, high EVM window position\n\n<7_MErr_RMSlowLimCheck>\n limit check result\nMagnitude error RMS value, low EVM window position\n\n<8_MErr_RMShighLimCheck>\n limit check result\nMagnitude error RMS value, high EVM window position\n\n<9_MErrPeakLowLimCheck>\n limit check result\nMagnitude error peak value, low EVM window 
